vi "Extract from Start and End Index.vi"(8 "Error":errorcluster, 9 "End Index\n(-1) Last Point":i32, 10 "Start Index":i32, 11 "WavBuf":refnum<class "WavBuf.lvclass">) -> (0 "Error Out":errorcluster, 1 "End Out":i32, 2 "Start Out":i32, 3 "Buffer Out":T1)   [LabVIEW 2025, in "WavBuf.lvclass"]
uses:
  WavBuf.lvclass
  Universal Controls/Waveform_Data.ctl
  WavBuf.lvclass/WavBuf.ctl
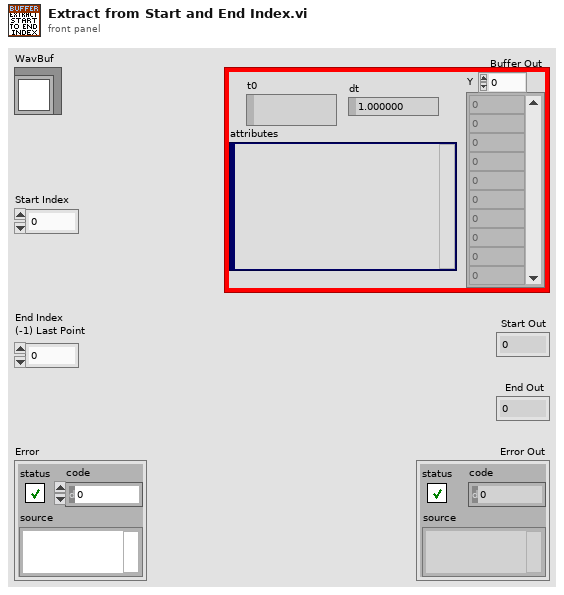
[diagram p1: front panel]
types:
  T1 = typedef "Waveform_Data.ctl" = waveform(dbl)
  T2 = typedef "Ref_DVR_Buffer.ctl" = refnum<data-value>
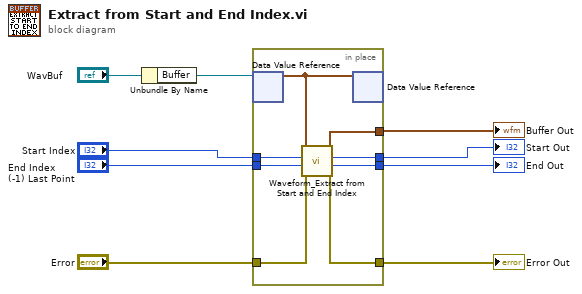
[diagram p0: block diagram]
diagram:
  n1 = Unbundle By Name("WavBuf") -> ("Buffer"=w1:T2)
  n2 = in-place {
    in-place-border: "Error" -> [w17]
    in-place-border: [w16] -> w8
    in-place-border: "Start Index" -> [w15]
    in-place-border: "End Index\n(-1) Last Point" -> [w14]
    in-place-border: [w13] -> w7
    in-place-border: [w12] -> w6
    in-place-border: [w11] -> w5
    n3 = in-place-dvr #1(w1) -> (w10:T1)  [unwired: 1 out]
    n4 = call "Waveform_Extract from Start and End Index.vi"("Error"=w17, "End Index\n(-1) Last point"=w14, "Start Index"=w15, "Raw Data Waveform"=w10) -> ("Error Out"=w16:errorcluster, "End Out"=w11:i32, "Start Out"=w12:i32, "Waveform Out"=w13:T1)  [unwired: 4 out]
    n5 = in-place-dvr #1(w10) -> ()  [unwired: 2 out]
  }
  "Error Out" <- w8
  "Buffer Out" <- w7
  "Start Out" <- w6
  "End Out" <- w5
